vi "FMSweep-Check Parameters.vi"(0 "FMSweep":T1, 11 "error in (no error)":errorcluster) -> (15 "error out":errorcluster)   [LabVIEW 2020]
uses:
  FM Sweep Params.ctl
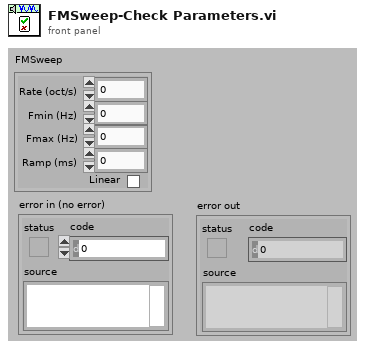
[diagram p1: front panel]
types:
  T1 = typedef "FM Sweep Params.ctl" = cluster{"Rate (oct/s)":dbl, "Fmin (Hz)":dbl, "Fmax (Hz)":dbl, "Ramp (ms)":dbl, "Linear":bool}
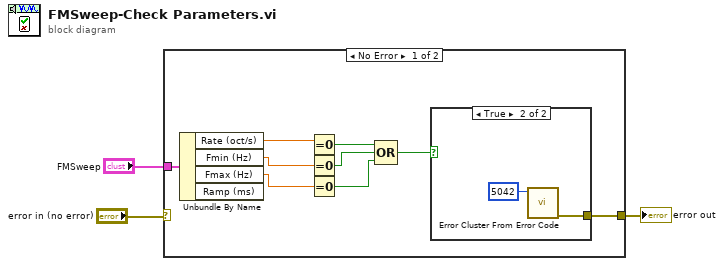
[diagram p0: block diagram]
diagram:
  n1 = case shown="No Error" "error in (no error)" {
    selector: "error in (no error)" -> [_ w15]
    tunnel: [w4 w15] -> w2
    tunnel: "FMSweep" -> [w12 _]
    frame No Error {
      n2 = Unbundle By Name(w12) -> ("Rate (oct/s)"=w11:dbl, "Fmin (Hz)"=w10:dbl, "Fmax (Hz)"=w9:dbl)  [unwired: 1 out]
      n3 = Equal To 0?(x=w11) -> (x = 0?=w8:bool)
      n4 = Equal To 0?(x=w10) -> (x = 0?=w7:bool)
      n5 = Equal To 0?(x=w9) -> (x = 0?=w6:bool)
      n6 = Compound Arithmetic op=OR(w8, w7, w6) -> (w5:bool)
      n7 = case shown="True" w5 {
        tunnel: [_ w14] -> w4
        frame False {
        }
        frame True {
          n8 = call <vilib>:"Error Cluster From Error Code.vi"("error code (0)"=5042) -> ("error out"=w14:errorcluster)  [unwired: 8 in]
        }
      }
    }
    frame Error {
    }
  }
  "error out" <- w2
